vi "ShiftAnalyzer.vi"() -> ()   [LabVIEW 2012]
uses:
  dependencies/ImageReg/BinarizationParameters.ctl
  dependencies/ImageReg/Edge and object parameters.ctl
  dependencies/ImageReg/Gaussian blur parameters.ctl
  <vilib>/Utility/file.llb/Write To Spreadsheet File (DBL).vi
  <vilib>/vision/NI_Vision_Development_Module.lvlib
panel:
  out "Binary alignment":dbl[](graph)
  out "Edge alignment":dbl[](graph)
  out "Blur alignment":dbl[](graph)
  in  "Gaussian blur parameters":T1={"large sigma"=20.0, "small sigma"=4.0, "equalize?"=FALSE}
  in  "Edge and object Parameters":T2={"Canny Edge Parameters"={"Sigma"=1.0, "HThresh"=0.7, "LThres"=0.2, "WindowSize"=9}, "Smoothing parameters"={"X Size"=3, "Y Size"=3, "% Tolerance"=40}, "Dilation iteration"=1, "Object recognition parameters"={"Objects"=0, "Threshold"=128, "Reject Border"=FALSE, "Fill Holes"=FALSE, "Min Object Size"=FALSE, "Min Size"=3, "Max Object Size"=FALSE, "Max Size"=100, "Show Search Area"=FALSE, "Show Center"=TRUE, "Show Bounding Box"=TRUE}} {"Object recognition parameters"."Objects" items=["Bright Objects", "Dark Objects"]; "Object recognition parameters"."Threshold" min=1 max=999999999 step=1; "Object recognition parameters"."Max Size" min=1 max=999999999 step=1; "Object recognition parameters"."Min Size" min=1 max=999999999 step=1; "Canny Edge Parameters"."LThres" min=0 max=1 format="%.2f"; "Canny Edge Parameters"."HThresh" min=0 max=1 format="%.2f"; "Canny Edge Parameters"."Sigma" min=0 max=1 format="%.2f"}
  in  "Binarization parameters":T3={"threshold percentage"=95.0, "equalize?"=FALSE, "Method (clustering)"=0} {"Method (clustering)" items=["clustering", "entropy", "metric", "moments", "inter-class variance"]}
  in  "quality file":path
  in  "Y coordinate file":path
  in  "X coordinate file":path
  in  "images folder":path
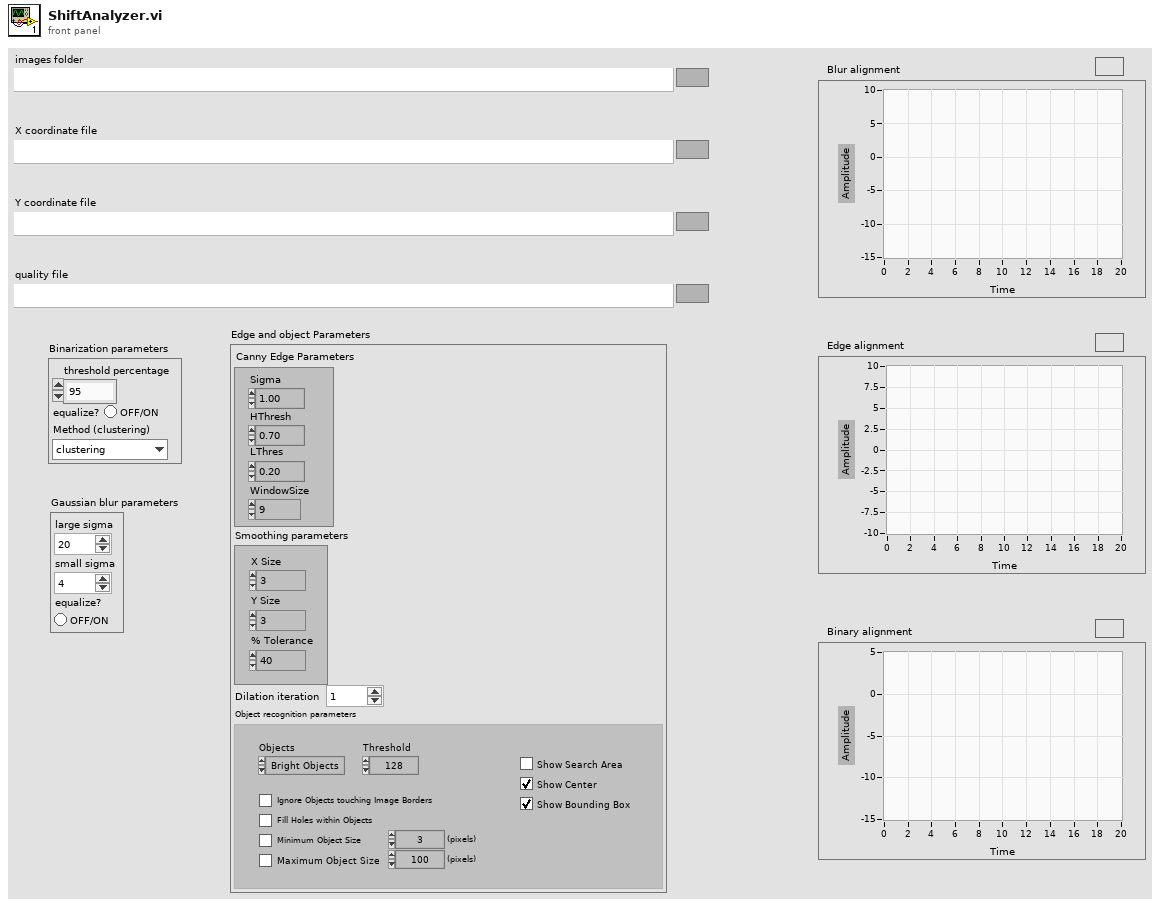
[diagram p1: front panel]
types:
  T1 = typedef "Gaussian blur parameters.ctl" = cluster{"large sigma":sgl, "small sigma":sgl, "equalize?":bool}
  T2 = typedef "Edge and object parameters.ctl" = cluster{"Canny Edge Parameters":cluster{"Sigma":sgl, "HThresh":sgl, "LThres":sgl, "WindowSize":i32}, "Smoothing parameters":cluster{"X Size":i32, "Y Size":i32, "% Tolerance":i32}, "Dilation iteration":i32, "Object recognition parameters":cluster{"Objects":u16, "Threshold":i32, "Reject Border":bool, "Fill Holes":bool, "Min Object Size":bool, "Min Size":i32, "Max Object Size":bool, "Max Size":i32, "Show Search Area":bool, "Show Center":bool, "Show Bounding Box":bool}}
  T3 = typedef "BinarizationParameters.ctl" = cluster{"threshold percentage":dbl, "equalize?":bool, "Method (clustering)":i32}
  T4 = typedef "Image Type" = u32
  T5 = typedef "IMAQ Image.ctl" = refnum<image>
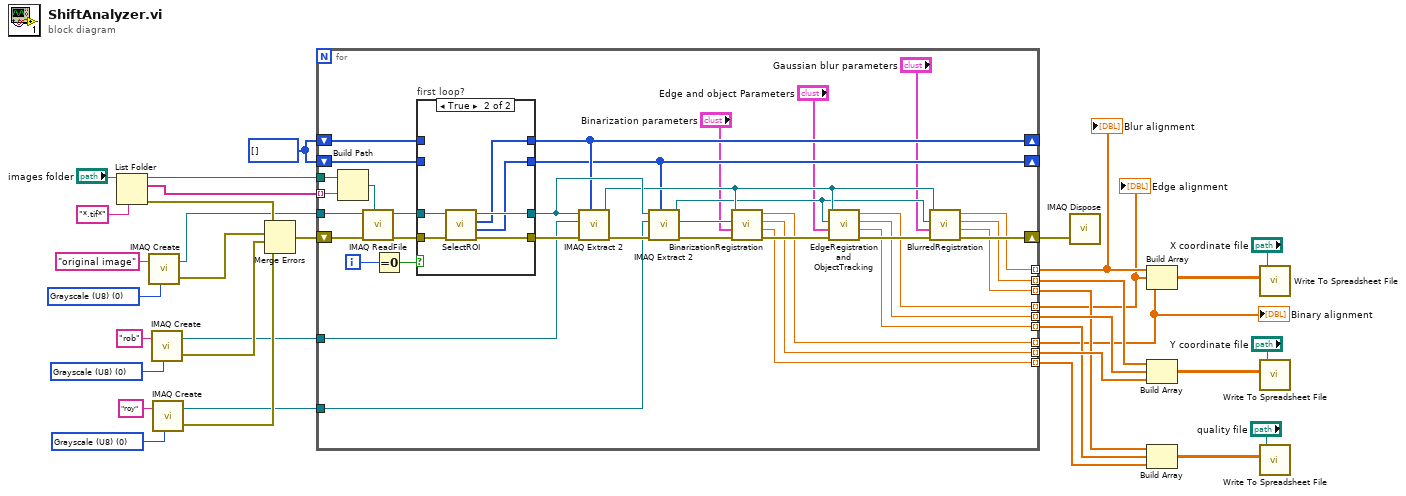
[diagram p0: block diagram]
diagram:
  w19 = i32[] [] ("Global Rectangle")
  w28 = T4 0 items=["Grayscale (U8)", "Grayscale (I16)", "Grayscale (SGL)", "Complex (CSG)", "RGB (U32)", "HSL (U32)", "RGB (U64)", "Grayscale (U16)"] ("Image Type")
  w29 = T4 0 items=["Grayscale (U8)", "Grayscale (I16)", "Grayscale (SGL)", "Complex (CSG)", "RGB (U32)", "HSL (U32)", "RGB (U64)", "Grayscale (U16)"] ("Image Type")
  w30 = T4 0 items=["Grayscale (U8)", "Grayscale (I16)", "Grayscale (SGL)", "Complex (CSG)", "RGB (U32)", "HSL (U32)", "RGB (U64)", "Grayscale (U16)"] ("Image Type")
  n1 = List Folder(path="images folder", pattern="*.tif*") -> (path out=w20:path, filenames=w27:string[], error out=w26:errorcluster)  [unwired: 2 in, 1 out]
  n2 = call "IMAQ Create"("Image Name"="original image", "Image Type"=w30) -> ("New Image"=w21:T5, "error out"=w25:errorcluster)  [unwired: 3 in]
  n3 = call "IMAQ Create"("Image Name"="rob", "Image Type"=w29) -> ("New Image"=w18:T5, "error out"=w24:errorcluster)  [unwired: 3 in]
  n4 = call "IMAQ Create"("Image Name"="roy", "Image Type"=w28) -> ("New Image"=w17:T5, "error out"=w23:errorcluster)  [unwired: 3 in]
  n5 = Merge Errors(w26, w25, w24, w23) -> (w22:errorcluster)
  n6 = for {
    tunnel: w27 -> [w67] mode=indexing
    shift-right: [w50] -> w4
    shift-left: w22 -> [w70]
    tunnel: w20 -> [w68]
    shift-right: [w52] -> _
    shift-left: w19 -> [w64]
    shift-right: [w51] -> _
    shift-left: w19 -> [w63]
    tunnel: w18 -> [w59]
    tunnel: w17 -> [w58]
    tunnel: w21 -> [w69]
    tunnel: [w49] -> w2 mode=indexing
    tunnel: [w48] -> w11 mode=indexing
    tunnel: [w47] -> w8 mode=indexing
    tunnel: [w46] -> w1 mode=indexing
    tunnel: [w45] -> w12 mode=indexing
    tunnel: [w44] -> w9 mode=indexing
    tunnel: [w43] -> w3 mode=indexing
    tunnel: [w42] -> w13 mode=indexing
    tunnel: [w41] -> w10 mode=indexing
    i -> [w65]
    n7 = Build Path(base path=w68, name or relative path=w67) -> (appended path=w71:path)
    n8 = call "IMAQ ReadFile"("File Path"=w71, "error in (no error)"=w70, "Image"=w69) -> ("error out"=w36:errorcluster, "Image Out"=w37:T5)  [unwired: 4 in, 3 out]
    n9 = Equal To 0?(x=w65) -> (x = 0?=w66:bool)
    n10 = case "first loop?" shown="True" w66 {
      tunnel: w36 -> [w73 w81]
      tunnel: w37 -> [w74 w79]
      tunnel: [w73 w80] -> w62
      tunnel: [w74 w78] -> w60
      tunnel: [w75 w76] -> w51
      tunnel: [w72 w77] -> w52
      tunnel: w63 -> [w75 _]
      tunnel: w64 -> [w72 _]
      frame False {
      }
      frame True {
        n11 = call "SelectROI.vi"("error in (no error)"=w81, "Image in"=w79) -> ("error out"=w80:errorcluster, "Global Rectangle Roy"=w76:i32[], "Global Rectangle Rob"=w77:i32[], "Image out"=w78:T5)  [unwired: 6 in]
      }
    }
    n12 = call "IMAQ Extract 2"("Optional Rectangle"=w52, "error in (no error)"=w62, "Image Dst"=w59, "Image Src"=w60) -> ("error out"=w61:errorcluster, "Image Dst Out"=w54:T5)  [unwired: 6 in]
    n13 = call "IMAQ Extract 2"("Optional Rectangle"=w51, "error in (no error)"=w61, "Image Dst"=w58, "Image Src"=w60) -> ("error out"=w57:errorcluster, "Image Dst Out"=w53:T5)  [unwired: 6 in]
    n14 = call "BinarizationRegistration.vi"("error in"=w57, "Binarization parameters"="Binarization parameters", "Roy"=w53, "Rob"=w54) -> ("error out"=w56:errorcluster, "quality"=w47:dbl, "y translation"=w48:dbl, "x translation"=w49:dbl)  [unwired: 4 in]
    n15 = call "EdgeRegistration and ObjectTracking.vi"("error in (no error)"=w56, "Edge and object Parameters"="Edge and object Parameters", "Roy"=w53, "Rob"=w54) -> ("error out"=w55:errorcluster, "Max value"=w44:dbl, "y translation"=w45:dbl, "x translation"=w46:dbl)  [unwired: 2 in, 2 out]
    n16 = call "BlurredRegistration.vi"("error in"=w55, "Gaussian blur parameters"="Gaussian blur parameters", "roy"=w53, "rob"=w54) -> ("error out"=w50:errorcluster, "alignment quality"=w41:dbl, "y displacement"=w42:dbl, "x displacement"=w43:dbl)  [unwired: 4 in]
  }
  "Blur alignment" <- w3
  "Edge alignment" <- w1
  "Binary alignment" <- w2
  n17 = call "IMAQ Dispose"("error in (no error)"=w4) -> ()  [unwired: 5 in, 1 out]
  n18 = Build Array(w3, w1, w2) -> (w16:dbl[][])
  n19 = Build Array(w13, w12, w11) -> (w15:dbl[][])
  n20 = Build Array(w10, w9, w8) -> (w14:dbl[][])
  n21 = call-poly <vilib>:"Write To Spreadsheet File.vi"("2D data"=w16, "file path (dialog if empty)"="X coordinate file") -> ()  [unwired: 6 in, 1 out]
  n22 = call-poly <vilib>:"Write To Spreadsheet File.vi"("2D data"=w15, "file path (dialog if empty)"="Y coordinate file") -> ()  [unwired: 6 in, 1 out]
  n23 = call-poly <vilib>:"Write To Spreadsheet File.vi"("2D data"=w14, "file path (dialog if empty)"="quality file") -> ()  [unwired: 6 in, 1 out]
